vi "project folder.vi"(9 "Project Info":T1, 11 "User folder Path":path) -> (2 "Project folder":path, 3 "Project folder":string)   [LabVIEW 2011]
uses:
  Project inputs.ctl
  AguaClara Library.lvlib
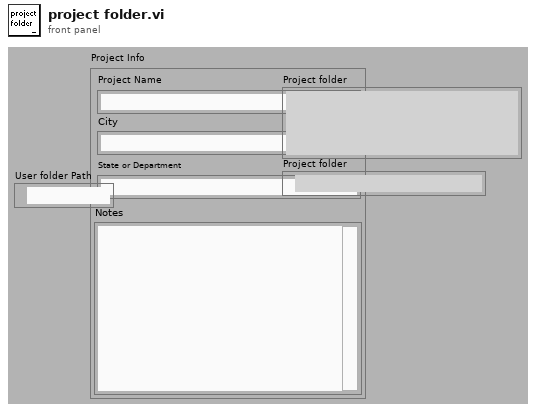
[diagram p1: front panel]
types:
  T1 = typedef "AguaClara Library.lvlib/Project inputs.ctl" = cluster{"Project Name":string, "City":string, "State":string, "Notes":string}
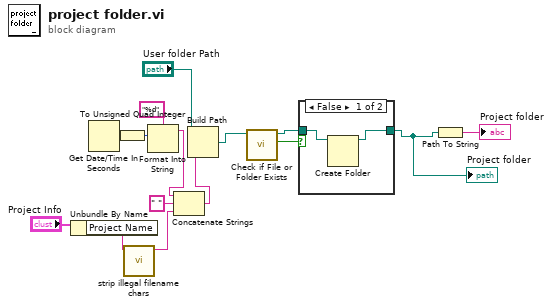
[diagram p0: block diagram]
diagram:
  n1 = Unbundle By Name("Project Info") -> ("Project Name"=w5:string)
  n2 = Get Date/Time In Seconds() -> (seconds since 1Jan1904=w13:timestamp)
  n3 = To Unsigned Quad Integer(1:w13) -> (0:w14:u64)
  n4 = call "strip illegal filename chars.vi"("string in"=w5) -> ("string out"=w1:string)  [unwired: 10 in]
  n5 = Format Into String(format string="%d", w14) -> (resulting string=w6:string)  [unwired: 2 in, 1 out]
  n6 = Concatenate Strings(w6, " " ("string"), w1) -> (w3:string)
  n7 = Build Path(base path="User folder Path", name or relative path=w3) -> (appended path=w9:path)
  n8 = call <vilib>:"Check if File or Folder Exists.vi"("path"=w9) -> ("file or folder exists?"=w10:bool, "dup path"=w11:path)  [unwired: 8 in, 1 out]
  n9 = case shown="False" w10 {
    tunnel: w11 -> [w17 w18]
    tunnel: [w16 w18] -> w2
    frame False {
      n10 = Create Folder(path (use dialog)=w17) -> (created path=w16:path)  [unwired: 2 in, 2 out]
    }
    frame True {
    }
  }
  "Project folder" <- w2
  n11 = Path To String(path=w2) -> (string=→"Project folder":string)
